vi "CUDA Toolkit Not Complex Process.vi"(11 "X size":i32=16384) -> (3 "Culab Time":dbl=1.016902899999991)   [LabVIEW 2020]
uses:
  Cuda/Source/Methods/Memory Control/SGL/CreateTensor&HTD(1DArraySGL).vi
  Cuda/Source/Tensor.lvclass
  <vilib>/Ngene/CuLab - GPU Accelerated Toolkit/Toolkit/Low_Level/Tensor_Classes/T_Children/T0D/T0D_Children/T0D_SGL/T0D_SGL.lvclass
  <vilib>/Analysis/NI_AALBase.lvlib
panel:
  out "Dest out":sgl=7.867303e+19
  in  "nb_loop":i32=6
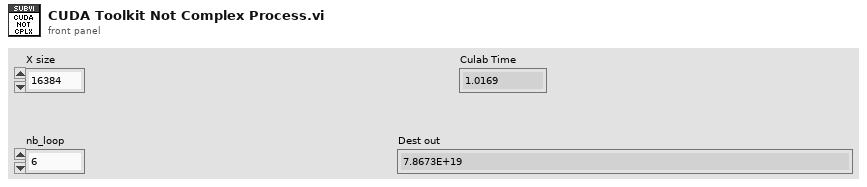
[diagram p1: front panel]
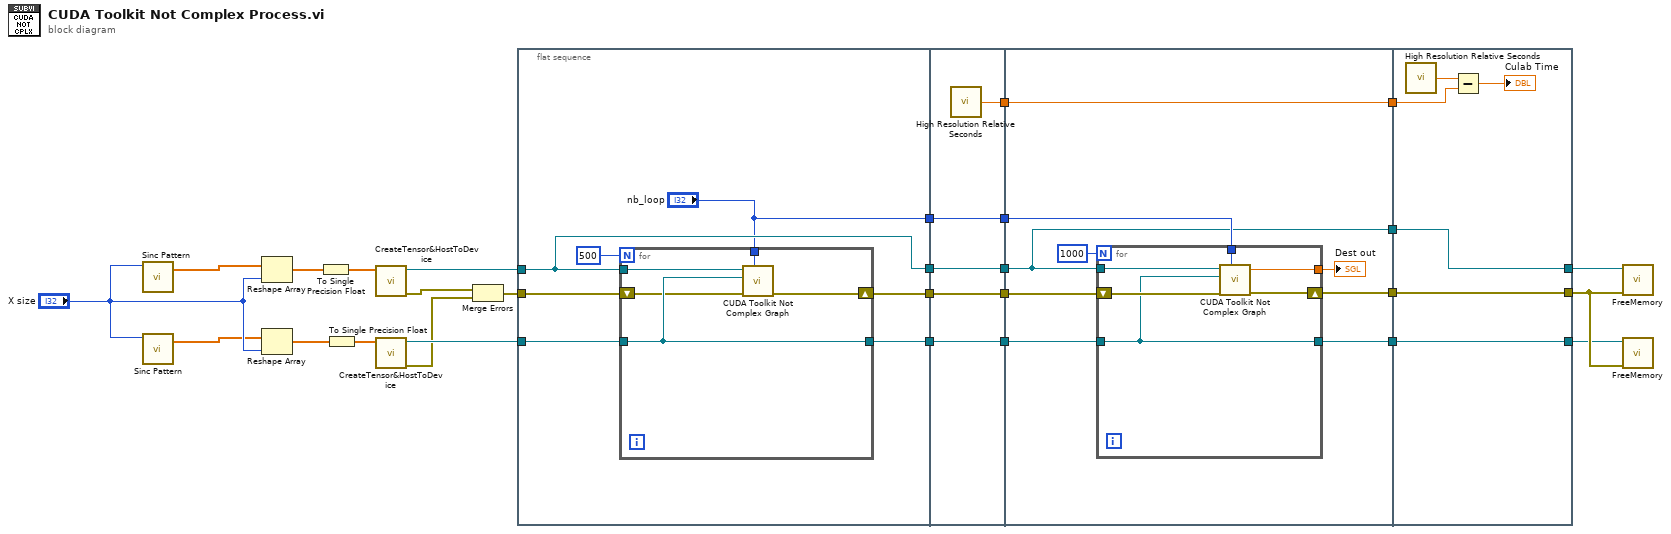
[diagram p0: block diagram]
diagram:
  n1 = call <vilib>:"Sinc Pattern.vi"("samples"="X size") -> ("Sinc Pattern"=w15:dbl[])  [unwired: 3 in, 1 out]
  n2 = call <vilib>:"Sinc Pattern.vi"("samples"="X size") -> ("Sinc Pattern"=w14:dbl[])  [unwired: 3 in, 1 out]
  n3 = Reshape Array(w15, "X size") -> (w18:dbl[])
  n4 = Reshape Array(w14, "X size") -> (w17:dbl[])
  n5 = To Single Precision Float(number=w18) -> (single precision float=w13:sgl[])
  n6 = To Single Precision Float(number=w17) -> (single precision float=w11:sgl[])
  n7 = call-poly "CreateTensor&HostToDevice.vi"("data"=w13) -> ("error out"=w8:errorcluster, "Tensor out"=w12:refnum<class "Tensor.lvclass">)  [unwired: 9 in]
  n8 = call-poly "CreateTensor&HostToDevice.vi"("data"=w11) -> ("error out"=w9:errorcluster, "Tensor out"=w10:refnum<class "Tensor.lvclass">)  [unwired: 9 in]
  n9 = Merge Errors(w8, w9) -> (w16:errorcluster)
  n10 = flat-sequence {
    tunnel: w10 -> [w35]
    tunnel: w12 -> [w34]
    tunnel: [w34] -> w25
    tunnel: [w32] -> w23
    tunnel: ["nb_loop"] -> w20
    tunnel: w16 -> [w30]
    tunnel: [w29] -> w6
    tunnel: [w45] -> w28
    tunnel: [w44] -> w27
    tunnel: w25 -> [w44]
    tunnel: [w43] -> w24
    tunnel: w23 -> [w43]
    tunnel: [w42] -> w21
    tunnel: w20 -> [w42]
    tunnel: [w41] -> w7
    tunnel: w6 -> [w41]
    tunnel: w28 -> [w54]
    tunnel: [w54] -> w26
    tunnel: w27 -> [w47]
    tunnel: w24 -> [w53]
    tunnel: [w51] -> w22
    tunnel: w21 -> [w50]
    tunnel: w7 -> [w48]
    tunnel: [w47] -> w5
    tunnel: [w46] -> w2
    tunnel: w26 -> [w65]
    tunnel: [w63] -> w3
    tunnel: w22 -> [w63]
    tunnel: w5 -> [w62]
    tunnel: [w62] -> w4
    tunnel: w2 -> [w61]
    tunnel: [w61] -> w1
    frame #0 {
      n11 = for {
        N: 500 -> [_]
        tunnel: w35 -> [w39]
        tunnel: w34 -> [w40]
        tunnel: [w39] -> w32
        tunnel: "nb_loop" -> [w38]
        shift-right: [w36] -> w29
        shift-left: w30 -> [w37]
        n12 = call "CUDA Toolkit Not Complex Graph.vi"("nb_loop"=w38, "error in (no error)"=w37, "B"=w39, "A"=w40) -> ("error out"=w36:errorcluster)  [unwired: 6 in, 1 out]
      }
    }
    frame #1 {
      n13 = call <vilib>:"High Resolution Relative Seconds.vi"() -> ("relative seconds"=w45:dbl)
    }
    frame #2 {
      n14 = for {
        N: 1000 -> [_]
        tunnel: w53 -> [w55]
        tunnel: [w57] -> w49
        tunnel: w47 -> [w60]
        tunnel: w50 -> [w59]
        tunnel: [w55] -> w46
        shift-right: [w56] -> w51
        shift-left: w48 -> [w58]
        n15 = call "CUDA Toolkit Not Complex Graph.vi"("nb_loop"=w59, "error in (no error)"=w58, "B"=w55, "A"=w60) -> ("error out"=w56:errorcluster, "sum"=w57:sgl)  [unwired: 6 in]
      }
      "Dest out" <- w49
    }
    frame #3 {
      n16 = call <vilib>:"High Resolution Relative Seconds.vi"() -> ("relative seconds"=w66:dbl)
      n17 = Subtract(x=w66, y=w65) -> (x-y=→"Culab Time":dbl)
    }
  }
  n18 = call "FreeMemory.vi"("error in"=w3, "Tensor in"=w4) -> ()  [unwired: 9 in, 1 out]
  n19 = call "FreeMemory.vi"("error in"=w3, "Tensor in"=w1) -> ()  [unwired: 9 in, 1 out]
